vi "IsEmpty.vi"(11 "POTTypedCircularBuffer in":refnum<class "ErrorLogBuffer.lvclass">) -> (2 "Empty?":bool, 3 "POTTypedCircularBuffer out":refnum<class "ErrorLogBuffer.lvclass">)   [LabVIEW 2024, in "ErrorLogBuffer.lvclass"]
uses:
  ErrorLogBuffer.lvclass
  ErrorLogBuffer.lvclass/ErrorLogBuffer.ctl
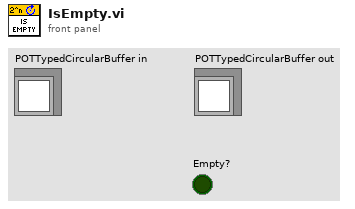
[diagram p1: front panel]
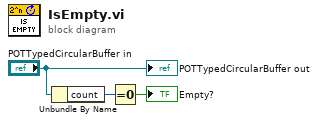
[diagram p0: block diagram]
diagram:
  n1 = Unbundle By Name("POTTypedCircularBuffer in") -> ("count"=w2:i32)
  n2 = Equal To 0?(x=w2) -> (x = 0?=→"Empty?":bool)
  "POTTypedCircularBuffer out" <- "POTTypedCircularBuffer in"
